vi "Datasheet Statistics Result.vi"(6 "Connection Refnum":T1, 8 "error in (no error)":errorcluster, 10 "Statistics Results":T3, 11 "Query Parameters":T5) -> (0 "error out":errorcluster, 1 "columns":i32, 2 "FORM":bool, 3 "Keyed Array":T2)   [LabVIEW 2011]
uses:
  Datasheet Analysis Parameters.ctl
  Statistics Data.ctl
  CGI SimpleStat Results.ctl
  ITK EXT/utils/keyedarr.llb/Keyed Array.ctl
  Summitek EXT/ODBC/SQL Controls/Connection Refnum.ctl
  ITK EXT/utils/strutil.llb/Case Matching.ctl
panel:
  out "Frequency Array":dbl[](array[numeric]) format="%#_14g"
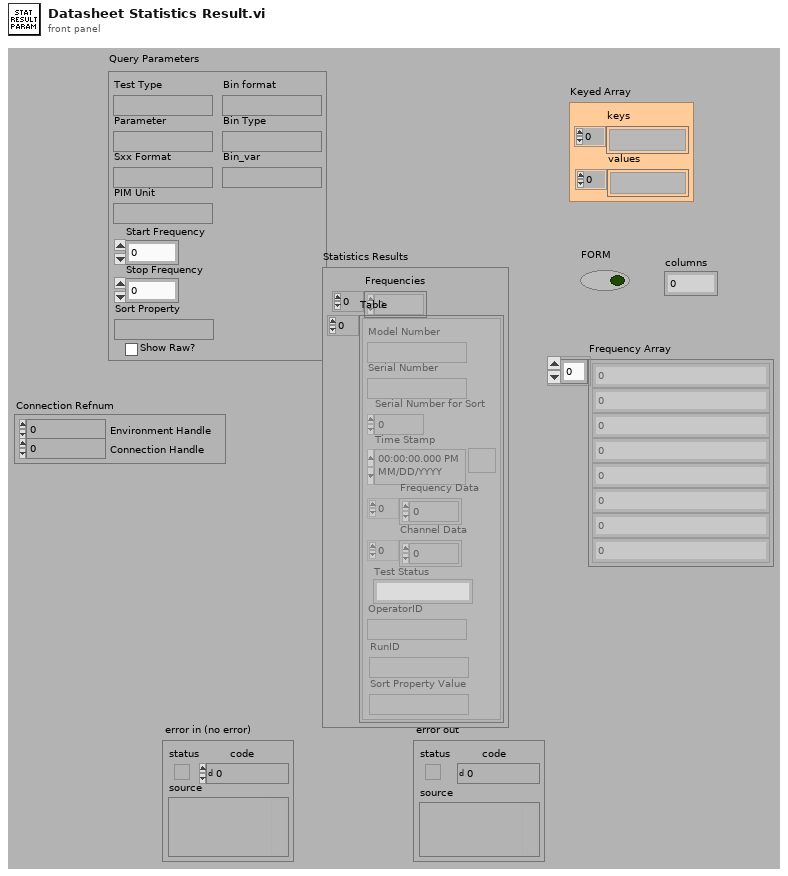
[diagram p1: front panel]
types:
  T1 = typedef "Connection Refnum.ctl" = cluster{"Environment Handle":i32, "Connection Handle":i32}
  T2 = typedef "Keyed Array.ctl" = cluster{"keys":string[], "values":string[]}
  T3 = typedef "Statistics Data.ctl" = cluster{"Table":T4[], "Frequencies":dbl[]}
  T4 = typedef "CGI SimpleStat Results.ctl" = cluster{"Model Number":string, "Serial Number for Sort":i32, "Serial Number":string, "Time Stamp":timestamp, "Channel Data":dbl[], "Test Status":string, "OperatorID":string, "Frequency Data":dbl[], "RunID":string, "Sort Property Value":string}
  T5 = typedef "Datasheet Analysis Parameters.ctl" = cluster{"Test Type":string, "Parameter":string, "Sxx Format":string, "PIM Unit":string, "Start Frequency":dbl, "Stop Frequency":dbl, "Sort Property":string, "Show Raw?":bool, "Bin format":string, "Bin Type":string, "Bin_var":string}
  T6 = typedef "Case Matching.ctl" = enum16{"a != A", "a == A", "system"}
  T7 = enum16{"Log MAG", "Lin MAG", "VSWR", "Phase", "Delay", "Insertion Loss", "Isolation", "Return Loss"}
  T8 = typedef "Field Record.ctl" = cluster{"ixField":i32, "iSequenceOrder":i32, "sxFieldId":string, "sxSequenceId":string, "sDisplayName":string, "sValue":string, "sUnits":string, "nDataType":T9, "nNextItem":T10, "fSystem":bool, "fSystemValue":bool, "fRequired":bool, "fSetAtTest":bool, "fTestField":bool, "fDeleted":bool, "fIndexed":bool, "fFreeList":bool}
  T9 = typedef "Field DataTypes.ctl" = enum32{"text", "numeric", "list", "timestamp", "boolean"}
  T10 = typedef "Field NextItem.ctl" = enum32{"Reset", "Retain", "Auto-Increment"}
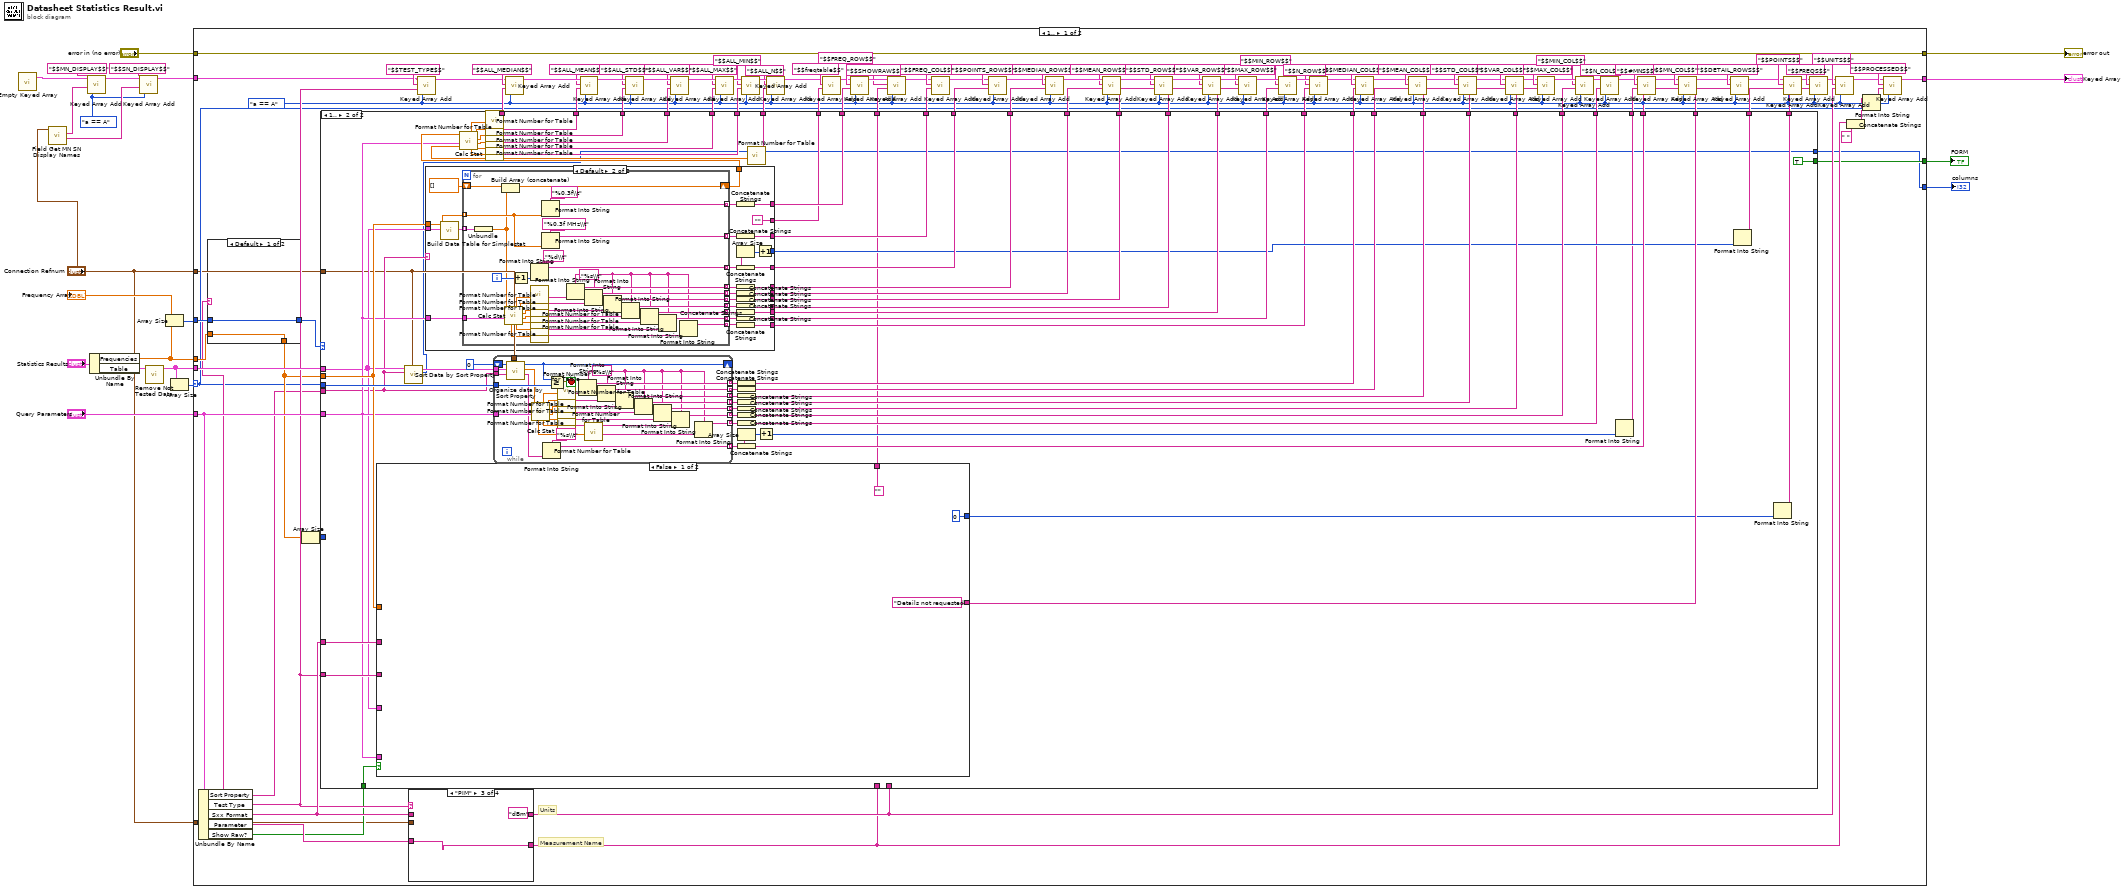
[diagram p0: block diagram]
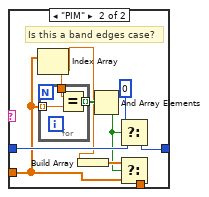
[diagram p2: hidden frame]
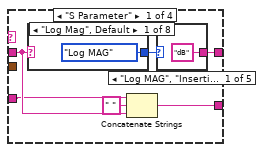
[diagram p3: hidden frame]
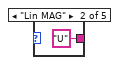
[diagram p4: hidden frame]
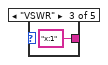
[diagram p5: hidden frame]
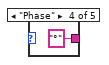
[diagram p6: hidden frame]
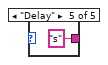
[diagram p7: hidden frame]
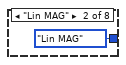
[diagram p8: hidden frame]
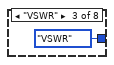
[diagram p9: hidden frame]
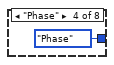
[diagram p10: hidden frame]
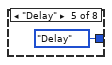
[diagram p11: hidden frame]
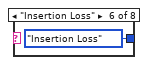
[diagram p12: hidden frame]
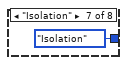
[diagram p13: hidden frame]
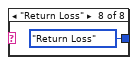
[diagram p14: hidden frame]
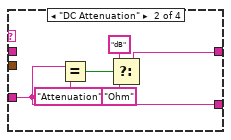
[diagram p15: hidden frame]
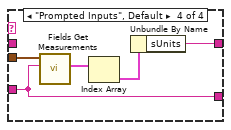
[diagram p16: hidden frame]
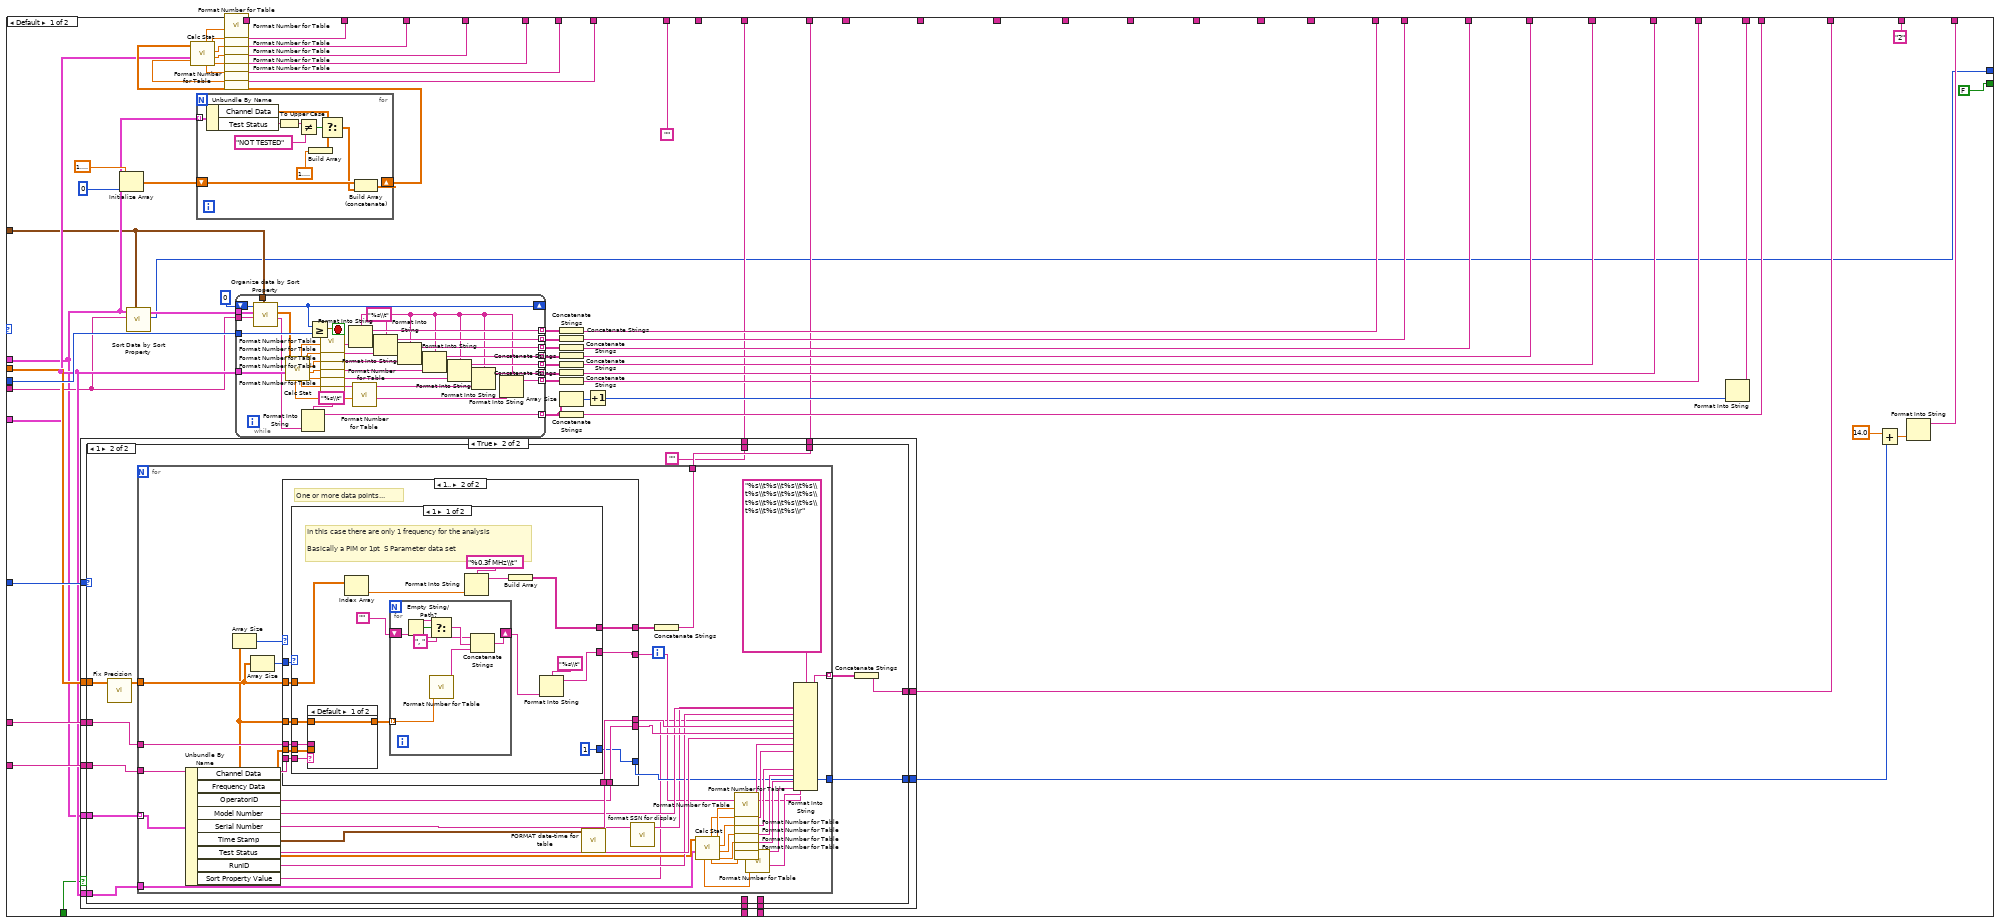
[diagram p17: hidden frame]
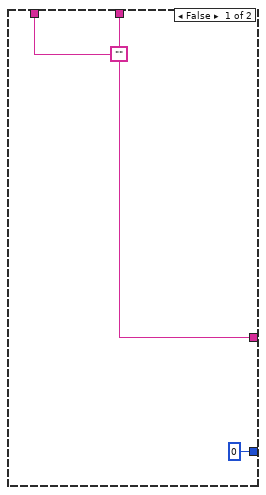
[diagram p18: hidden frame]
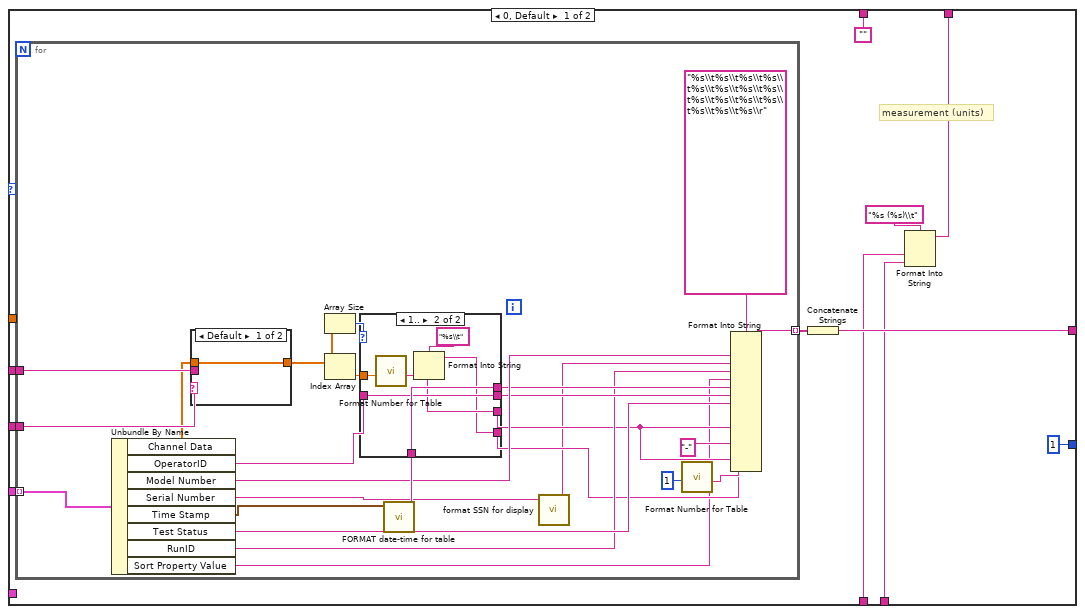
[diagram p19: hidden frame]
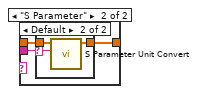
[diagram p20: hidden frame]
diagram:
  w5 = Case_Matching."a == A" ("case matching (sensitive)")
  n1 = call "Empty Keyed Array.vi"() -> ("empty keyed array"=w4:T2)  [unwired: 3 out]
  n2 = call "Field Get MN SN Display Names.vi"("Connection Refnum"="Connection Refnum") -> ("Serial Number Display Name"=w7:string, "Model Number Display Name"=w8:string)  [unwired: 1 in, 8 out]
  n3 = call "Keyed Array Add.vi"("case matching (sensitive)"=w5, "value"=w8, "key"="$$MN_DISPLAY$$", "array in"=w4) -> ("array out"=w9:T2)  [unwired: 3 out]
  n4 = Unbundle By Name("Statistics Results") -> ("Frequencies"=w15:dbl[], "Table"=w14:T4[])
  "Frequency Array" <- w15
  n5 = call "Keyed Array Add.vi"("case matching (sensitive)"=w5, "value"=w7, "key"="$$SN_DISPLAY$$", "array in"=w9) -> ("array out"=w6:T2)  [unwired: 3 out]
  n6 = call "Remove Not Tested Data.vi"("Table"=w14) -> ("Table 2"=w13:T4[])  [unwired: 10 out]
  n7 = Array Size(array=w15) -> (size(s)=w18:i32)
  n8 = Array Size(array=w13) -> (size(s)=w16:i32)
  n9 = case shown="1.." w16 {
    selector: w16 -> [w29 w775]
    tunnel: [w65 w801] -> w21
    tunnel: "error in (no error)" -> [w65 w801]
    tunnel: [w31 w777] -> w12
    tunnel: w18 -> [w61 w798]
    tunnel: "Query Parameters" -> [w130 w841]
    tunnel: w15 -> [w58 w797]
    tunnel: w13 -> [w131 _]
    tunnel: w6 -> [w35 w781]
    tunnel: "Connection Refnum" -> [w25 _]
    tunnel: "Connection Refnum" -> [w24 w770]
    tunnel: [w23 FALSE] -> w2
    tunnel: [w22 0] -> w1
    frame 1.. {
      w30 = Case_Matching."a == A" ("case matching (sensitive)")
      # "Measurement Name"
      # "Units"
      n10 = Unbundle By Name(w130) -> ("Sort Property"=w41:string, "Test Type"=w56:string, "Sxx Format"=w135:string, "Parameter"=w136:string, "Show Raw?"=w40:bool)
      n11 = case shown="Default" w56 {
        tunnel: w61 -> [w147 w156]
        tunnel: [w147 w155] -> w60
        tunnel: [w146 w152] -> w55
        tunnel: w58 -> [w146 w151]
        frame Default {
        }
        frame "PIM" {
          # "Is this a band edges case?"
          n12 = Index Array(array=w151) -> (element=w148:dbl)  [unwired: 1 in]
          n13 = for {
            tunnel: w148 -> [w159]
            tunnel: w151 -> [w158] mode=indexing
            tunnel: [w157] -> w150 mode=indexing
            n14 = Equal?(x=w159, y=w158) -> (x = y?=w157:bool)
          }
          n15 = Build Array(w148) -> (w153:dbl[])
          n16 = And Array Elements(Boolean array=w150) -> (logical AND=w149:bool)
          n17 = Select(t=0, s=w149, f=w156) -> (s? t:f=w155:i32)
          n18 = Select(t=w153, s=w149, f=w151) -> (s? t:f=w152:dbl[])
        }
      }
      n19 = Array Size(array=w55) -> (size(s)=w59:i32)
      n20 = case shown="\"PIM\"" w56 {
        tunnel: w135 -> [w162 _ _ _]
        tunnel: w136 -> [w160 w179 w185 w188]
        tunnel: [w164 w180 "dBm" ("search string") w189] -> w42
        tunnel: [w161 w179 w185 w188] -> w28
        tunnel: w24 -> [_ _ _ w187]
        frame "S Parameter" {
          n21 = case shown="\"Log Mag\", Default" w162 {
            tunnel: [T7."Log MAG" ("Display Format") T7."Lin MAG" ("Display Format") T7."VSWR" ("Display Format") T7."Phase" ("Display Format") T7."Delay" ("Display Format") T7."Insertion Loss" ("Display Format") T7."Isolation" ("Display Format") T7."Return Loss" ("Display Format")] -> w165
            frame "Log Mag", Default {
            }
            frame "Lin MAG" {
            }
            frame "VSWR" {
            }
            frame "Phase" {
            }
            frame "Delay" {
            }
            frame "Insertion Loss" {
            }
            frame "Isolation" {
            }
            frame "Return Loss" {
            }
          }
          n22 = Concatenate Strings(w160, " " ("search string"), w162) -> (w161:string)
          n23 = case shown="\"Log MAG\", \"Insertion Loss\"..\"Return Loss\", Default" w165 {
            tunnel: ["dB" "U" "x:1" "°" "s"] -> w164
            frame "Log MAG", "Insertion Loss".."Return Loss", Default {
            }
            frame "Lin MAG" {
            }
            frame "VSWR" {
            }
            frame "Phase" {
            }
            frame "Delay" {
            }
          }
        }
        frame "DC Attenuation" {
          n24 = Equal?(x=w179, y="Attenuation" ("search string")) -> (x = y?=w183:bool)
          n25 = Select(t="dB" ("search string"), s=w183, f="Ohm" ("search string")) -> (s? t:f=w180:string)
        }
        frame "PIM" {
        }
        frame "Prompted Inputs", Default {
          n26 = call "Fields Get Measurements.vi"("sDisplayName (empty, get all)"=w188, "Connection Refnum"=w187) -> ("Measurement Fields"=w191:T8[])  [unwired: 9 out]
          n27 = Index Array(array=w191) -> (element=w190:T8)  [unwired: 1 in]
          n28 = Unbundle By Name(w190) -> ("sUnits"=w189:string)
        }
      }
      n29 = case shown="1.." w60 {
        tunnel: w55 -> [w211 w506]
        tunnel: w131 -> [w198 w498]
        tunnel: w56 -> [w225 w551]
        tunnel: w135 -> [w226 w552]
        tunnel: w29 -> [w234 w553]
        tunnel: w130 -> [w210 w505]
        tunnel: [w233 w550] -> w129
        tunnel: [w232 w543] -> w128
        tunnel: [w231 w542] -> w125
        tunnel: [w229 w541] -> w124
        tunnel: [w228 w540] -> w123
        tunnel: [w227 w539] -> w122
        tunnel: [w230 w538] -> w121
        tunnel: [w247 w530] -> w107
        tunnel: [w246 w529] -> w106
        tunnel: [w245 w528] -> w105
        tunnel: [w244 w527] -> w104
        tunnel: [w243 w526] -> w103
        tunnel: [w242 w525] -> w102
        tunnel: [_ w524] -> w90
        tunnel: [_ w523] -> w89
        tunnel: [_ w522] -> w88
        tunnel: [_ w521] -> w87
        tunnel: [_ w520] -> w86
        tunnel: [_ w519] -> w85
        tunnel: [_ w518] -> w84
        tunnel: [_ w517] -> w82
        tunnel: [w224 w516] -> w77
        tunnel: w28 -> [w213 _]
        tunnel: [w208 w514] -> w71
        tunnel: ["2" w513] -> w70
        tunnel: [w220 w508] -> w67
        tunnel: ["" w494] -> w62
        tunnel: w59 -> [w214 _]
        tunnel: [w212 w507] -> w57
        tunnel: [w204 w503] -> w52
        tunnel: [_ w502] -> w47
        tunnel: [w202 w500] -> w44
        tunnel: w42 -> [w201 _]
        tunnel: w41 -> [w199 w495]
        tunnel: w40 -> [w197 w497]
        tunnel: [w196 w496] -> w37
        tunnel: w25 -> [w195 w493]
        tunnel: [FALSE TRUE] -> w23
        tunnel: [w192 w491] -> w22
        frame Default {
          n30 = case shown="True" w197 {
            tunnel: w226 -> [_ w267]
            tunnel: w225 -> [_ w266]
            tunnel: [w254 w265] -> w224
            tunnel: w214 -> [_ w264]
            tunnel: w213 -> [_ w263]
            tunnel: [w254 w262] -> w212
            tunnel: w211 -> [_ w261]
            tunnel: w210 -> [_ w260]
            tunnel: [0 w259] -> w206
            tunnel: w201 -> [_ w258]
            tunnel: w198 -> [_ w257]
            tunnel: [w254 w256] -> w196
            frame False {
              w254 = ""
            }
            frame True {
              n31 = case shown="1" w264 {
                tunnel: w257 -> [w278 w330]
                tunnel: w267 -> [w277 w328]
                tunnel: w266 -> [w276 w329]
                tunnel: [w274 w326] -> w265
                tunnel: w261 -> [_ w324]
                tunnel: [w272 w325] -> w262
                tunnel: w263 -> [w271 _]
                tunnel: w260 -> [_ w321]
                tunnel: [1 w322] -> w259
                tunnel: w258 -> [w269 _]
                tunnel: ["" ""] -> w256
                frame 0, Default {
                  # "measurement (units)"
                  n32 = for {
                    tunnel: w278 -> [w303] mode=indexing
                    tunnel: w276 -> [w298]
                    tunnel: w277 -> [w297]
                    tunnel: [w290] -> w275 mode=indexing
                    w287 = "-" ("search string")
                    n33 = Unbundle By Name(w303) -> ("Channel Data"=w296:dbl[], "OperatorID"=w295:string, "Model Number"=w293:string, "Serial Number"=w282:string, "Time Stamp"=w279:timestamp, "Test Status"=w294:string, "RunID"=w289:string, "Sort Property Value"=w280:string)
                    n34 = case shown="Default" w298 {
                      tunnel: [w304 w306] -> w299
                      tunnel: w297 -> [_ w305]
                      tunnel: w296 -> [w304 w307]
                      frame Default {
                      }
                      frame "S Parameter" {
                        n35 = case shown="Default" w305 {
                          selector: w305 -> [_ w309]
                          tunnel: w307 -> [w308 w311]
                          tunnel: [w308 w310] -> w306
                          frame "delay" {
                          }
                          frame Default {
                            n36 = call "S Parameter Unit Convert.vi"("Format"=w309, "Waveform IN"=w311) -> ("Waveform out"=w310:dbl[])  [unwired: 1 in, 8 out]
                          }
                        }
                      }
                    }
                    n37 = Array Size(array=w299) -> (size(s)=w302:i32)
                    n38 = Index Array(array=w299) -> (element=w301:dbl)  [unwired: 1 in]
                    n39 = call "FORMAT date-time for table.vi"("Time Stamp"=w279) -> ("String"=w300:string)  [unwired: 1 in, 9 out]
                    n40 = case shown="1.." w302 {
                      tunnel: [w312 w315] -> w284
                      tunnel: w301 -> [_ w317]
                      tunnel: w300 -> [_ w319]
                      tunnel: [w312 w319] -> w292
                      tunnel: [w312 w318] -> w291
                      tunnel: w295 -> [_ w318]
                      tunnel: ["Not Tested\\t" ("search string") w314] -> w283
                      frame 0, Default {
                        w312 = "-" ("search string")
                      }
                      frame 1.. {
                        n41 = call "Format Number for Table.vi"("Number"=w317) -> ("Number String"=w315:string)  [unwired: 2 in, 8 out]
                        n42 = Format Into String(format string="%s\\t", w315) -> (resulting string=w314:string)  [unwired: 2 in, 1 out]
                      }
                    }
                    n43 = call "format SSN for display.vi"("string"=w282) -> ("s? t:f"=w281:string)  [unwired: 4 out]
                    n44 = call "Format Number for Table.vi"("Number"=1) -> ("Number String"=w285:string)  [unwired: 2 in, 8 out]
                    n45 = Format Into String(format string="%s\\t%s\\t%s\\t%s\\t%s\\t%s\\t%s\\t%s\\t%s\\t%s\\t%s\\t%s\\t%s\\t%s\\t%s\\r", w293, w281, w289, w280, w292, w291, w294, w284, w284, w287, w287, w284, w284, w285, w283) -> (resulting string=w290:string)  [unwired: 2 in, 1 out]
                  }
                  n46 = Concatenate Strings(w275) -> (w274:string)
                  n47 = Format Into String(format string="%s (%s)\\t" ("search string"), w271, w269) -> (resulting string=w272:string)  [unwired: 2 in, 1 out]
                }
                frame 1 {
                  n48 = call "Fix Precision.vi"("DBL"=w324) -> ("DBLOut"=w323:dbl[])  [unwired: 10 out]
                  n49 = for {
                    tunnel: w330 -> [w370] mode=indexing
                    tunnel: w323 -> [w355]
                    tunnel: w329 -> [w367]
                    tunnel: w328 -> [w366]
                    tunnel: [w362] -> w327 mode=indexing
                    tunnel: [w339] -> w322
                    tunnel: [w357] -> w325
                    tunnel: w321 -> [w333]
                    n50 = Unbundle By Name(w370) -> ("Channel Data"=w346:dbl[], "Frequency Data"=w361:dbl[], "OperatorID"=w359:string, "Model Number"=w360:string, "Serial Number"=w335:string, "Time Stamp"=w331:timestamp, "Test Status"=w363:string, "RunID"=w358:string, "Sort Property Value"=w332:string)
                    n51 = Array Size(array=w346) -> (size(s)=w369:i32)
                    n52 = Array Size(array=w355) -> (size(s)=w354:i32)
                    n53 = call "FORMAT date-time for table.vi"("Time Stamp"=w331) -> ("String"=w368:string)  [unwired: 1 in, 9 out]
                    n54 = case shown="1.." w369 {
                      tunnel: w346 -> [_ w389]
                      tunnel: ["Not Tested" ("search string") w390] -> w365
                      tunnel: w368 -> [_ w390]
                      tunnel: w355 -> [w376 w383]
                      tunnel: w367 -> [_ w388]
                      tunnel: w366 -> [_ w387]
                      tunnel: w359 -> [_ w386]
                      tunnel: [w374 w386] -> w364
                      tunnel: w361 -> [_ w385]
                      tunnel: [_ w384] -> w356
                      tunnel: w354 -> [_ w382]
                      tunnel: [w373 w381] -> w336
                      tunnel: [w371 w380] -> w339
                      frame Default {
                        w374 = "-" ("search string")
                        # "This is no data case"
                        n55 = for {
                          tunnel: w376 -> [_] mode=indexing
                          tunnel: w374 -> [w377]
                          tunnel: [w378] -> w372 mode=indexing
                          n56 = Format Into String(format string="%s\\t", w377) -> (resulting string=w378:string)  [unwired: 2 in, 1 out]
                        }
                        n57 = Array Size(array=w372) -> (size(s)=w371:i32)
                        n58 = Concatenate Strings(w372) -> (w373:string)
                      }
                      frame 1.. {
                        # "One or more data points..."
                        n59 = case shown="1" w382 {
                          tunnel: w389 -> [w405 w428]
                          tunnel: w388 -> [w404 w427]
                          tunnel: w387 -> [w403 w426]
                          tunnel: w385 -> [w402 w422]
                          tunnel: [w397 w425] -> w384
                          tunnel: w383 -> [w400 w423]
                          tunnel: [w396 w420] -> w381
                          tunnel: [1 w418] -> w380
                          frame 1 {
                            # "In this case there are only 1 frequency for the analysis   \n\nBasically a PIM or 1pt  S Parameter data set"
                            n60 = case shown="Default" w404 {
                              tunnel: w405 -> [w413 w417]
                              tunnel: [w413 w416] -> w393
                              tunnel: w403 -> [_ w415]
                              tunnel: w402 -> [_ w414]
                              frame Default {
                              }
                              frame "S Parameter" {
                                n61 = call "S Parameter Unit Convert.vi"("Frequency Array"=w414, "Format"=w415, "Waveform IN"=w417) -> ("Waveform out"=w416:dbl[])  [unwired: 8 out]
                              }
                            }
                            n62 = Index Array(array=w400) -> (element=w399:dbl)  [unwired: 1 in]
                            n63 = for {
                              shift-right: [w411] -> w392
                              shift-left: "" -> [w407]
                              tunnel: w393 -> [w406] mode=indexing
                              n64 = Empty String/Path?(string/path=w407) -> (empty?=w410:bool)
                              n65 = Select(t=w407, s=w410, f=", " ("format string")) -> (s? t:f=w408:string)
                              n66 = call "Format Number for Table.vi"("Number"=w406) -> ("Number String"=w412:string)  [unwired: 2 in, 8 out]
                              n67 = Concatenate Strings(w407, w408, w412) -> (w411:string)
                            }
                            n68 = Format Into String(format string="%0.3f MHz\\t" ("search string"), w399) -> (resulting string=w398:string)  [unwired: 2 in, 1 out]
                            n69 = Build Array(w398) -> (w397:string[])
                            n70 = Format Into String(format string="%s\\t", w392) -> (resulting string=w396:string)  [unwired: 2 in, 1 out]
                          }
                          frame Default {
                            # "For this case, like PI.weight.  There are no Frequencies"
                            n71 = case shown="Default" w427 {
                              tunnel: w428 -> [w429 w433]
                              tunnel: [w429 w432] -> w424
                              tunnel: w426 -> [_ w431]
                              tunnel: w422 -> [_ w430]
                              frame Default {
                              }
                              frame "S Parameter" {
                                n72 = call "S Parameter Unit Convert.vi"("Frequency Array"=w430, "Format"=w431, "Waveform IN"=w433) -> ("Waveform out"=w432:dbl[])  [unwired: 8 out]
                              }
                            }
                            n73 = call "Fix Precision.vi"("DBL"=w422) -> ("DBLOut"=w421:dbl[])  [unwired: 10 out]
                            n74 = for {
                              tunnel: [w439] -> w419 mode=indexing
                              tunnel: w423 -> [w435] mode=indexing
                              tunnel: w421 -> [_]
                              tunnel: w424 -> [w444]
                              tunnel: [w434] -> w425 mode=indexing
                              i -> [w437]
                              n75 = Less Than 0?(x=w437) -> (x < 0?=w445:bool)
                              n76 = Index Array(array=w444, index=w437) -> (element=w443:dbl)
                              n77 = Select(t=1.1447298858494002, s=w445, f=w443) -> (s? t:f=w442:dbl)
                              n78 = Format Into String(format string="%0.3f MHz\\t" ("search string"), w435) -> (resulting string=w434:string)  [unwired: 2 in, 1 out]
                              n79 = call "Format Number for Table.vi"("Number"=w442) -> ("Number String"=w440:string)  [unwired: 2 in, 8 out]
                              n80 = Format Into String(format string="%s\\t", w440) -> (resulting string=w439:string)  [unwired: 2 in, 1 out]
                            }
                            n81 = Concatenate Strings(w419) -> (w420:string)
                            n82 = Array Size(array=w419) -> (size(s)=w418:i32)
                          }
                        }
                      }
                    }
                    n83 = call "format SSN for display.vi"("string"=w335) -> ("s? t:f"=w334:string)  [unwired: 4 out]
                    n84 = Concatenate Strings(w356) -> (w357:string)
                    n85 = call "Calc Stat.vi"("Query Parameters"=w333, "Channel Data"=w346) -> ("Maximum"=w348:dbl, "Variance"=w349:dbl, "Standard Deviation"=w350:dbl, "Mean"=w352:dbl, "Minimum"=w347:dbl, "Median"=w351:dbl, "N"=w338:dbl)  [unwired: 2 in, 1 out]
                    n86 = call "Format Number for Table.vi"("Number"=w352) -> ("Number String"=w345:string)  [unwired: 2 in, 8 out]
                    n87 = call "Format Number for Table.vi"("Number"=w351) -> ("Number String"=w344:string)  [unwired: 2 in, 8 out]
                    n88 = call "Format Number for Table.vi"("Number"=w350) -> ("Number String"=w343:string)  [unwired: 2 in, 8 out]
                    n89 = call "Format Number for Table.vi"("Number"=w349) -> ("Number String"=w342:string)  [unwired: 2 in, 8 out]
                    n90 = call "Format Number for Table.vi"("Number"=w348) -> ("Number String"=w341:string)  [unwired: 2 in, 8 out]
                    n91 = call "Format Number for Table.vi"("Number"=w347) -> ("Number String"=w340:string)  [unwired: 2 in, 8 out]
                    n92 = call "Format Number for Table.vi"("Number"=w338) -> ("Number String"=w337:string)  [unwired: 2 in, 8 out]
                    n93 = Format Into String(format string="%s\\t%s\\t%s\\t%s\\t%s\\t%s\\t%s\\t%s\\t%s\\t%s\\t%s\\t%s\\t%s\\t%s\\t%s\\r", w360, w334, w358, w332, w365, w364, w363, w345, w344, w343, w342, w341, w340, w337, w336) -> (resulting string=w362:string)  [unwired: 2 in, 1 out]
                  }
                  n94 = Concatenate Strings(w327) -> (w326:string)
                }
              }
            }
          }
          n95 = Initialize Array(1.1447298858494002, 0 ("dimension size")) -> (w218:dbl[])
          n96 = call "Sort Data by Sort Property.vi"("Connection Refnum"=w195, "Sort Property Name"=w199, "Table"=w198) -> ("Numeric"=w192:i32, "Table 2"=w200:T4[])  [unwired: 1 in, 6 out]
          n97 = for {
            tunnel: w198 -> [w490] mode=indexing
            shift-right: [w482] -> w215
            shift-left: w218 -> [w484]
            n98 = Unbundle By Name(w490) -> ("Channel Data"=w487:dbl[], "Test Status"=w489:string)
            n99 = To Upper Case(1:w489) -> (0:w480:string)
            n100 = Not Equal?(x=w480, y="NOT TESTED" ("key")) -> (x != y?=w488:bool)
            n101 = Build Array(1.1447298858494002) -> (w486:dbl[])
            n102 = Select(t=w487, s=w488, f=w486) -> (s? t:f=w483:dbl[])
            n103 = Build Array (concatenate)(w484, w483) -> (w482:dbl[])
          }
          n104 = call "Calc Stat.vi"("Query Parameters"=w210, "Channel Data"=w215) -> ("Maximum"=w248:dbl, "Variance"=w250:dbl, "Standard Deviation"=w251:dbl, "Mean"=w252:dbl, "Minimum"=w249:dbl, "Median"=w253:dbl, "N"=w205:dbl)  [unwired: 2 in, 1 out]
          n105 = call "Format Number for Table.vi"("Number"=w253) -> ("Number String"=w247:string)  [unwired: 2 in, 8 out]
          n106 = call "Format Number for Table.vi"("Number"=w252) -> ("Number String"=w246:string)  [unwired: 2 in, 8 out]
          n107 = call "Format Number for Table.vi"("Number"=w251) -> ("Number String"=w245:string)  [unwired: 2 in, 8 out]
          n108 = call "Format Number for Table.vi"("Number"=w250) -> ("Number String"=w244:string)  [unwired: 2 in, 8 out]
          n109 = call "Format Number for Table.vi"("Number"=w248) -> ("Number String"=w243:string)  [unwired: 2 in, 8 out]
          n110 = call "Format Number for Table.vi"("Number"=w249) -> ("Number String"=w242:string)  [unwired: 2 in, 8 out]
          n111 = call "Format Number for Table.vi"("Number"=w205) -> ("Number String"=w204:string)  [unwired: 2 in, 8 out]
          n112 = while {
            shift-right: [w446] -> _
            shift-left: 0 -> [w479]
            tunnel: w200 -> [w478]
            tunnel: w234 -> [w477]
            tunnel: w210 -> [w474]
            tunnel: [w465] -> w221 mode=indexing
            tunnel: [w463] -> w240 mode=indexing
            tunnel: [w457] -> w239 mode=indexing
            tunnel: [w456] -> w238 mode=indexing
            tunnel: [w455] -> w237 mode=indexing
            tunnel: [w454] -> w236 mode=indexing
            tunnel: [w453] -> w235 mode=indexing
            tunnel: [w449] -> w203 mode=indexing
            tunnel: w199 -> [w448]
            tunnel: w195 -> [w447]
            stop <- w476 stop-if-true
            w452 = "%s\\t" ("format string")
            n113 = call "Organize data by Sort Property.vi"("Connection Refnum"=w447, "Sort Property Name"=w448, "Table"=w478, "Start Index"=w479) -> ("Property Value"=w467:string, "Channel Data"=w475:dbl[], "End Index"=w446:i32)  [unwired: 1 in, 4 out]
            n114 = call "Calc Stat.vi"("Query Parameters"=w474, "Channel Data"=w475) -> ("Maximum"=w473:dbl, "Variance"=w471:dbl, "Standard Deviation"=w470:dbl, "Mean"=w469:dbl, "Minimum"=w472:dbl, "Median"=w468:dbl, "N"=w451:dbl)  [unwired: 2 in, 1 out]
            n115 = Format Into String(format string="%s\\t", w467) -> (resulting string=w465:string)  [unwired: 2 in, 1 out]
            n116 = Greater Or Equal?(x=w446, y=w477) -> (x >= y?=w476:bool)
            n117 = call "Format Number for Table.vi"("Number"=w468) -> ("Number String"=w464:string)  [unwired: 2 in, 8 out]
            n118 = call "Format Number for Table.vi"("Number"=w469) -> ("Number String"=w462:string)  [unwired: 2 in, 8 out]
            n119 = call "Format Number for Table.vi"("Number"=w470) -> ("Number String"=w461:string)  [unwired: 2 in, 8 out]
            n120 = call "Format Number for Table.vi"("Number"=w471) -> ("Number String"=w460:string)  [unwired: 2 in, 8 out]
            n121 = call "Format Number for Table.vi"("Number"=w473) -> ("Number String"=w459:string)  [unwired: 2 in, 8 out]
            n122 = call "Format Number for Table.vi"("Number"=w472) -> ("Number String"=w458:string)  [unwired: 2 in, 8 out]
            n123 = Format Into String(format string=w452, w464) -> (resulting string=w463:string)  [unwired: 2 in, 1 out]
            n124 = call "Format Number for Table.vi"("Number"=w451) -> ("Number String"=w450:string)  [unwired: 2 in, 8 out]
            n125 = Format Into String(format string=w452, w462) -> (resulting string=w457:string)  [unwired: 2 in, 1 out]
            n126 = Format Into String(format string=w452, w461) -> (resulting string=w456:string)  [unwired: 2 in, 1 out]
            n127 = Format Into String(format string=w452, w460) -> (resulting string=w455:string)  [unwired: 2 in, 1 out]
            n128 = Format Into String(format string=w452, w459) -> (resulting string=w454:string)  [unwired: 2 in, 1 out]
            n129 = Format Into String(format string=w452, w458) -> (resulting string=w453:string)  [unwired: 2 in, 1 out]
            n130 = Format Into String(format string=w452, w450) -> (resulting string=w449:string)  [unwired: 2 in, 1 out]
          }
          n131 = Concatenate Strings(w240) -> (w232:string)
          n132 = Concatenate Strings(w239) -> (w231:string)
          n133 = Concatenate Strings(w238) -> (w230:string)
          n134 = Concatenate Strings(w237) -> (w229:string)
          n135 = Concatenate Strings(w236) -> (w228:string)
          n136 = Concatenate Strings(w235) -> (w227:string)
          n137 = Concatenate Strings(w203) -> (w202:string)
          n138 = Array Size(array=w221) -> (size(s)=w222:i32)
          n139 = Concatenate Strings(w221) -> (w233:string)
          n140 = Increment(x=w222) -> (x+1=w219:i32)
          n141 = Format Into String(w219) -> (resulting string=w220:string)  [unwired: 3 in, 1 out]
          n142 = Add(x=14.0, y=w206) -> (x+y=w209:dbl)
          n143 = Format Into String(w209) -> (resulting string=w208:string)  [unwired: 3 in, 1 out]
        }
        frame 1.. {
          n144 = case shown="False" w497 {
            tunnel: w552 -> [_ w643]
            tunnel: w551 -> [_ w642]
            tunnel: ["Details not requested" w640] -> w516
            tunnel: [0 w637] -> w515
            tunnel: w506 -> [_ w636]
            tunnel: w505 -> [_ w635]
            tunnel: w498 -> [_ w634]
            tunnel: ["" ""] -> w496
            frame False {
            }
            frame True {
              n145 = for {
                tunnel: w634 -> [w682] mode=indexing
                tunnel: w636 -> [w654]
                tunnel: w642 -> [w679]
                tunnel: w643 -> [w678]
                tunnel: [w673] -> w641 mode=indexing
                tunnel: [w669] -> w639
                tunnel: w635 -> [w667]
                # "ALL Frequency"
                # "P/F"
                # "Operator"
                # "time"
                # "Run"
                # "SN"
                # "MN"
                # "Need to extract array that represents the repeated points in the PIM sweep\nand show the maximum."
                n146 = Unbundle By Name(w682) -> ("Channel Data"=w668:dbl[], "Frequency Data"=w672:dbl[], "OperatorID"=w671:string, "Model Number"=w648:string, "Serial Number"=w649:string, "Time Stamp"=w644:timestamp, "Test Status"=w674:string, "RunID"=w646:string, "Sort Property Value"=w645:string)
                n147 = call "Fix Precision.vi"("DBL"=w654) -> ("DBLOut"=w653:dbl[])  [unwired: 10 out]
                n148 = Array Size(array=w668) -> (size(s)=w681:i32)
                n149 = call "FORMAT date-time for table.vi"("Time Stamp"=w644) -> ("String"=w680:string)  [unwired: 1 in, 9 out]
                n150 = case shown="1.." w681 {
                  tunnel: w668 -> [_ w697]
                  tunnel: [w685 w699] -> w670
                  tunnel: ["Not Tested" ("search string") w698] -> w676
                  tunnel: w680 -> [_ w698]
                  tunnel: w653 -> [w686 w693]
                  tunnel: w679 -> [_ w696]
                  tunnel: w678 -> [_ w695]
                  tunnel: w671 -> [_ w694]
                  tunnel: [w683 w694] -> w675
                  tunnel: w672 -> [_ w691]
                  frame 0, Default {
                    w683 = "-" ("search string")
                    n151 = for {
                      tunnel: w686 -> [_] mode=indexing
                      tunnel: w683 -> [w687]
                      tunnel: [w688] -> w685 mode=indexing
                      n152 = Format Into String(format string="%s\\t", w687) -> (resulting string=w688:string)  [unwired: 2 in, 1 out]
                    }
                  }
                  frame 1.. {
                    n153 = case shown="\"S Parameter\"" w696 {
                      tunnel: w697 -> [w700 w704]
                      tunnel: [w700 w703] -> w692
                      tunnel: w695 -> [_ w702]
                      tunnel: w691 -> [_ w701]
                      frame Default {
                      }
                      frame "S Parameter" {
                        n154 = call "S Parameter Unit Convert.vi"("Frequency Array"=w701, "Format"=w702, "Waveform IN"=w704) -> ("Waveform out"=w703:dbl[])  [unwired: 8 out]
                      }
                    }
                    n155 = call "Fix Precision.vi"("DBL"=w691) -> ("DBLOut"=w690:dbl[])  [unwired: 10 out]
                    n156 = for {
                      tunnel: [w708] -> w699 mode=indexing
                      tunnel: w693 -> [w711] mode=indexing
                      tunnel: w690 -> [w712]
                      tunnel: w692 -> [w710]
                      n157 = while {
                        tunnel: w712 -> [w728]
                        tunnel: w711 -> [w727]
                        tunnel: w710 -> [w726]
                        shift-right: [w720] -> _
                        shift-left: 0 -> [w722]
                        shift-right: [w718] -> w705
                        shift-left: "" -> [w714]
                        stop <- w713 stop-if-true
                        n158 = Empty String/Path?(string/path=w714) -> (empty?=w717:bool)
                        n159 = Search 1D Array(1D array=w728, element=w727, start index (0)=w722) -> (index of element=w721:i32)
                        n160 = Less Than 0?(x=w721) -> (x < 0?=w713:bool)
                        n161 = Select(t=w714, s=w717, f=", " ("format string")) -> (s? t:f=w715:string)
                        n162 = Index Array(array=w726, index=w721) -> (element=w725:dbl)
                        n163 = Select(t=1.1447298858494002, s=w713, f=w725) -> (s? t:f=w724:dbl)
                        n164 = Increment(x=w721) -> (x+1=w720:i32)
                        n165 = call "Format Number for Table.vi"("Number"=w724) -> ("Number String"=w719:string)  [unwired: 2 in, 8 out]
                        n166 = case shown="True" w713 {
                          tunnel: w719 -> [w732 _]
                          tunnel: [w731 w733] -> w718
                          tunnel: w715 -> [w730 _]
                          tunnel: w714 -> [w729 w733]
                          frame False {
                            n167 = Concatenate Strings(w729, w730, w732) -> (w731:string)
                          }
                          frame True {
                          }
                        }
                      }
                      n168 = Format Into String(format string="%s\\t", w705) -> (resulting string=w708:string)  [unwired: 2 in, 1 out]
                    }
                  }
                }
                n169 = call "format SSN for display.vi"("string"=w649) -> ("s? t:f"=w647:string)  [unwired: 4 out]
                n170 = Array Size(array=w670) -> (size(s)=w669:i32)
                n171 = Concatenate Strings(w670) -> (w651:string)
                n172 = call "Calc Stat.vi"("Query Parameters"=w667, "Channel Data"=w668) -> ("Maximum"=w658:dbl, "Variance"=w660:dbl, "Standard Deviation"=w662:dbl, "Mean"=w666:dbl, "Minimum"=w656:dbl, "Median"=w664:dbl, "N"=w652:dbl)  [unwired: 2 in, 1 out]
                n173 = call "Format Number for Table.vi"("Number"=w666) -> ("Number String"=w665:string)  [unwired: 2 in, 8 out]
                n174 = call "Format Number for Table.vi"("Number"=w664) -> ("Number String"=w663:string)  [unwired: 2 in, 8 out]
                n175 = call "Format Number for Table.vi"("Number"=w662) -> ("Number String"=w661:string)  [unwired: 2 in, 8 out]
                n176 = call "Format Number for Table.vi"("Number"=w660) -> ("Number String"=w659:string)  [unwired: 2 in, 8 out]
                n177 = call "Format Number for Table.vi"("Number"=w658) -> ("Number String"=w657:string)  [unwired: 2 in, 8 out]
                n178 = call "Format Number for Table.vi"("Number"=w656) -> ("Number String"=w655:string)  [unwired: 2 in, 8 out]
                n179 = call "Format Number for Table.vi"("Number"=w652) -> ("Number String"=w650:string)  [unwired: 2 in, 8 out]
                n180 = Format Into String(format string="%s\\t%s\\t%s\\t%s\\t%s\\t%s\\t%s\\t%s\\t%s\\t%s\\t%s\\t%s\\t%s\\t%s\\t%s\\r", w648, w647, w646, w645, w676, w675, w674, w665, w663, w661, w659, w657, w655, w650, w651) -> (resulting string=w673:string)  [unwired: 2 in, 1 out]
              }
              n181 = Add(x=w639, y=14) -> (x+y=w637:i32)
              n182 = Concatenate Strings(w641) -> (w640:string)
            }
          }
          n183 = call "Sort Data by Sort Property.vi"("Connection Refnum"=w493, "Sort Property Name"=w495, "Table"=w498) -> ("Numeric"=w491:i32, "Table 2"=w499:T4[])  [unwired: 1 in, 6 out]
          n184 = case shown="Default" w495 {
            tunnel: [w561 w592] -> w531
            tunnel: [w555 w585] -> w524
            tunnel: [w555 w584] -> w523
            tunnel: [w555 w583] -> w522
            tunnel: [w555 w582] -> w521
            tunnel: [w555 w581] -> w520
            tunnel: [w555 w580] -> w519
            tunnel: [w555 w578] -> w518
            tunnel: [w555 w577] -> w517
            tunnel: [w559 w574] -> w512
            tunnel: [w557 w572] -> w507
            tunnel: w506 -> [w558 w571]
            tunnel: w505 -> [_ w569]
            tunnel: [w555 w567] -> w502
            tunnel: w498 -> [_ w566]
            tunnel: [w555 ""] -> w494
            frame "SPARA" {
              w559 = 0 ("dimension size")
              w555 = ""
              n185 = for {
                tunnel: w558 -> [w563] mode=indexing
                tunnel: [w562] -> w556 mode=indexing
                n186 = Format Into String(format string="%0.3f MHz\\t" ("search string"), w563) -> (resulting string=w562:string)  [unwired: 2 in, 1 out]
              }
              n187 = Initialize Array(0.0 ("dimension size"), w559) -> (w561:dbl[])
              n188 = Concatenate Strings(w556) -> (w557:string)
            }
            frame Default {
              n189 = call "Build Data Table for Simplestat.vi"("Table"=w566, "Frequency Array"=w571) -> ("All Data by Frequency"=w570:cluster{"Array":dbl[]}[])  [unwired: 1 in, 8 out]
              n190 = for {
                tunnel: w571 -> [w629] mode=indexing
                tunnel: [w624] -> w576 mode=indexing
                tunnel: w569 -> [w615]
                tunnel: [w622] -> w579 mode=indexing
                tunnel: [w623] -> w575 mode=indexing
                shift-right: [w625] -> w592
                shift-left: dbl[] [] -> [w626]
                tunnel: [w605] -> w591 mode=indexing
                tunnel: [w604] -> w590 mode=indexing
                tunnel: [w603] -> w589 mode=indexing
                tunnel: [w602] -> w588 mode=indexing
                tunnel: [w601] -> w587 mode=indexing
                tunnel: [w600] -> w586 mode=indexing
                tunnel: w570 -> [w599] mode=indexing
                tunnel: [w594] -> w568 mode=indexing
                i -> [w612]
                w597 = "%s\\t" ("format string")
                n191 = Unbundle(w599) -> ("Array"=w598:dbl[])
                n192 = Build Array (concatenate)(w626, w598) -> (w625:dbl[])
                n193 = call "Calc Stat.vi"("Query Parameters"=w615, "Channel Data"=w598) -> ("Maximum"=w616:dbl, "Variance"=w618:dbl, "Standard Deviation"=w619:dbl, "Mean"=w620:dbl, "Minimum"=w617:dbl, "Median"=w621:dbl, "N"=w595:dbl)  [unwired: 2 in, 1 out]
                n194 = Increment(x=w612) -> (x+1=w627:i32)
                n195 = Format Into String(format string="%d\\t" ("search string"), w627) -> (resulting string=w623:string)  [unwired: 2 in, 1 out]
                n196 = call "Format Number for Table.vi"("Number"=w621) -> ("Number String"=w611:string)  [unwired: 2 in, 8 out]
                n197 = call "Format Number for Table.vi"("Number"=w620) -> ("Number String"=w610:string)  [unwired: 2 in, 8 out]
                n198 = call "Format Number for Table.vi"("Number"=w619) -> ("Number String"=w609:string)  [unwired: 2 in, 8 out]
                n199 = call "Format Number for Table.vi"("Number"=w618) -> ("Number String"=w608:string)  [unwired: 2 in, 8 out]
                n200 = call "Format Number for Table.vi"("Number"=w616) -> ("Number String"=w607:string)  [unwired: 2 in, 8 out]
                n201 = call "Format Number for Table.vi"("Number"=w617) -> ("Number String"=w606:string)  [unwired: 2 in, 8 out]
                n202 = call "Format Number for Table.vi"("Number"=w595) -> ("Number String"=w596:string)  [unwired: 2 in, 8 out]
                n203 = Format Into String(format string="%0.3f\\t" ("search string"), w629) -> (resulting string=w622:string)  [unwired: 2 in, 1 out]
                n204 = Format Into String(format string="%0.3f MHz\\t" ("search string"), w629) -> (resulting string=w624:string)  [unwired: 2 in, 1 out]
                n205 = Format Into String(format string=w597, w611) -> (resulting string=w605:string)  [unwired: 2 in, 1 out]
                n206 = Format Into String(format string=w597, w610) -> (resulting string=w604:string)  [unwired: 2 in, 1 out]
                n207 = Format Into String(format string=w597, w609) -> (resulting string=w603:string)  [unwired: 2 in, 1 out]
                n208 = Format Into String(format string=w597, w608) -> (resulting string=w602:string)  [unwired: 2 in, 1 out]
                n209 = Format Into String(format string=w597, w607) -> (resulting string=w601:string)  [unwired: 2 in, 1 out]
                n210 = Format Into String(format string=w597, w606) -> (resulting string=w600:string)  [unwired: 2 in, 1 out]
                n211 = Format Into String(format string=w597, w596) -> (resulting string=w594:string)  [unwired: 2 in, 1 out]
              }
              n212 = Concatenate Strings(w579) -> (w578:string)
              n213 = Concatenate Strings(w576) -> (w572:string)
              n214 = Array Size(array=w575) -> (size(s)=w573:i32)
              n215 = Concatenate Strings(w575) -> (w577:string)
              n216 = Concatenate Strings(w591) -> (w585:string)
              n217 = Concatenate Strings(w590) -> (w584:string)
              n218 = Concatenate Strings(w589) -> (w583:string)
              n219 = Concatenate Strings(w588) -> (w582:string)
              n220 = Concatenate Strings(w587) -> (w581:string)
              n221 = Concatenate Strings(w586) -> (w580:string)
              n222 = Concatenate Strings(w568) -> (w567:string)
              n223 = Increment(x=w573) -> (x+1=w574:i32)
            }
          }
          n224 = call "Calc Stat.vi"("Query Parameters"=w505, "Channel Data"=w531) -> ("Maximum"=w532:dbl, "Variance"=w534:dbl, "Standard Deviation"=w535:dbl, "Mean"=w536:dbl, "Minimum"=w533:dbl, "Median"=w537:dbl, "N"=w504:dbl)  [unwired: 2 in, 1 out]
          n225 = call "Format Number for Table.vi"("Number"=w537) -> ("Number String"=w530:string)  [unwired: 2 in, 8 out]
          n226 = call "Format Number for Table.vi"("Number"=w536) -> ("Number String"=w529:string)  [unwired: 2 in, 8 out]
          n227 = call "Format Number for Table.vi"("Number"=w535) -> ("Number String"=w528:string)  [unwired: 2 in, 8 out]
          n228 = call "Format Number for Table.vi"("Number"=w534) -> ("Number String"=w527:string)  [unwired: 2 in, 8 out]
          n229 = call "Format Number for Table.vi"("Number"=w532) -> ("Number String"=w526:string)  [unwired: 2 in, 8 out]
          n230 = call "Format Number for Table.vi"("Number"=w533) -> ("Number String"=w525:string)  [unwired: 2 in, 8 out]
          n231 = while {
            shift-right: [w735] -> _
            shift-left: 0 -> [w767]
            tunnel: w499 -> [w766]
            tunnel: w553 -> [w765]
            tunnel: w505 -> [w762]
            tunnel: [w753] -> w510 mode=indexing
            tunnel: [w751] -> w549 mode=indexing
            tunnel: [w745] -> w548 mode=indexing
            tunnel: [w744] -> w547 mode=indexing
            tunnel: [w743] -> w546 mode=indexing
            tunnel: [w742] -> w545 mode=indexing
            tunnel: [w741] -> w544 mode=indexing
            tunnel: [w737] -> w501 mode=indexing
            tunnel: w495 -> [w736]
            tunnel: w493 -> [w734]
            stop <- w764 stop-if-true
            w740 = "%s\\t" ("format string")
            n232 = call "Organize data by Sort Property.vi"("Connection Refnum"=w734, "Sort Property Name"=w736, "Table"=w766, "Start Index"=w767) -> ("Property Value"=w755:string, "Channel Data"=w763:dbl[], "End Index"=w735:i32)  [unwired: 1 in, 4 out]
            n233 = call "Calc Stat.vi"("Query Parameters"=w762, "Channel Data"=w763) -> ("Maximum"=w761:dbl, "Variance"=w759:dbl, "Standard Deviation"=w758:dbl, "Mean"=w757:dbl, "Minimum"=w760:dbl, "Median"=w756:dbl, "N"=w739:dbl)  [unwired: 2 in, 1 out]
            n234 = Format Into String(format string="%s\\t", w755) -> (resulting string=w753:string)  [unwired: 2 in, 1 out]
            n235 = Greater Or Equal?(x=w735, y=w765) -> (x >= y?=w764:bool)
            n236 = call "Format Number for Table.vi"("Number"=w756) -> ("Number String"=w752:string)  [unwired: 2 in, 8 out]
            n237 = call "Format Number for Table.vi"("Number"=w757) -> ("Number String"=w750:string)  [unwired: 2 in, 8 out]
            n238 = call "Format Number for Table.vi"("Number"=w758) -> ("Number String"=w749:string)  [unwired: 2 in, 8 out]
            n239 = call "Format Number for Table.vi"("Number"=w759) -> ("Number String"=w748:string)  [unwired: 2 in, 8 out]
            n240 = call "Format Number for Table.vi"("Number"=w761) -> ("Number String"=w747:string)  [unwired: 2 in, 8 out]
            n241 = call "Format Number for Table.vi"("Number"=w760) -> ("Number String"=w746:string)  [unwired: 2 in, 8 out]
            n242 = Format Into String(format string=w740, w752) -> (resulting string=w751:string)  [unwired: 2 in, 1 out]
            n243 = call "Format Number for Table.vi"("Number"=w739) -> ("Number String"=w738:string)  [unwired: 2 in, 8 out]
            n244 = Format Into String(format string=w740, w750) -> (resulting string=w745:string)  [unwired: 2 in, 1 out]
            n245 = Format Into String(format string=w740, w749) -> (resulting string=w744:string)  [unwired: 2 in, 1 out]
            n246 = Format Into String(format string=w740, w748) -> (resulting string=w743:string)  [unwired: 2 in, 1 out]
            n247 = Format Into String(format string=w740, w747) -> (resulting string=w742:string)  [unwired: 2 in, 1 out]
            n248 = Format Into String(format string=w740, w746) -> (resulting string=w741:string)  [unwired: 2 in, 1 out]
            n249 = Format Into String(format string=w740, w738) -> (resulting string=w737:string)  [unwired: 2 in, 1 out]
          }
          n250 = Concatenate Strings(w549) -> (w543:string)
          n251 = Concatenate Strings(w548) -> (w542:string)
          n252 = Concatenate Strings(w547) -> (w538:string)
          n253 = Concatenate Strings(w546) -> (w541:string)
          n254 = Concatenate Strings(w545) -> (w540:string)
          n255 = Concatenate Strings(w544) -> (w539:string)
          n256 = Concatenate Strings(w501) -> (w500:string)
          n257 = Array Size(array=w510) -> (size(s)=w511:i32)
          n258 = Concatenate Strings(w510) -> (w550:string)
          n259 = call "Format Number for Table.vi"("Number"=w504) -> ("Number String"=w503:string)  [unwired: 2 in, 8 out]
          n260 = Increment(x=w511) -> (x+1=w509:i32)
          n261 = Format Into String(w509) -> (resulting string=w508:string)  [unwired: 3 in, 1 out]
          n262 = Format Into String(w512) -> (resulting string=w513:string)  [unwired: 3 in, 1 out]
          n263 = Format Into String(w515) -> (resulting string=w514:string)  [unwired: 3 in, 1 out]
        }
      }
      n264 = call "Keyed Array Add.vi"("case matching (sensitive)"=w30, "value"=w56, "key"="$$TEST_TYPE$$", "array in"=w35) -> ("array out"=w108:T2)  [unwired: 3 out]
      n265 = call "Keyed Array Add.vi"("case matching (sensitive)"=w30, "value"=w107, "key"="$$ALL_MEDIAN$$", "array in"=w108) -> ("array out"=w112:T2)  [unwired: 3 out]
      n266 = call "Keyed Array Add.vi"("case matching (sensitive)"=w30, "value"=w106, "key"="$$ALL_MEAN$$", "array in"=w112) -> ("array out"=w113:T2)  [unwired: 3 out]
      n267 = call "Keyed Array Add.vi"("case matching (sensitive)"=w30, "value"=w105, "key"="$$ALL_STD$$", "array in"=w113) -> ("array out"=w118:T2)  [unwired: 3 out]
      n268 = call "Keyed Array Add.vi"("case matching (sensitive)"=w30, "value"=w104, "key"="$$ALL_VAR$$", "array in"=w118) -> ("array out"=w119:T2)  [unwired: 3 out]
      n269 = call "Keyed Array Add.vi"("case matching (sensitive)"=w30, "value"=w103, "key"="$$ALL_MAX$$", "array in"=w119) -> ("array out"=w116:T2)  [unwired: 3 out]
      n270 = call "Keyed Array Add.vi"("case matching (sensitive)"=w30, "value"=w102, "key"="$$ALL_MIN$$", "array in"=w116) -> ("array out"=w54:T2)  [unwired: 3 out]
      n271 = call "Keyed Array Add.vi"("case matching (sensitive)"=w30, "value"=w52, "key"="$$ALL_N$$", "array in"=w54) -> ("array out"=w51:T2)  [unwired: 3 out]
      n272 = call "Keyed Array Add.vi"("value"=w62, "key"="$$freqtable$$", "array in"=w51) -> ("array out"=w64:T2)  [unwired: 1 in, 3 out]
      n273 = call "Keyed Array Add.vi"("case matching (sensitive)"=w30, "value"=w84, "key"="$$FREQ_ROW$$", "array in"=w64) -> ("array out"=w39:T2)  [unwired: 3 out]
      n274 = call "Keyed Array Add.vi"("case matching (sensitive)"=w30, "value"=w37, "key"="$$SHOWRAW$$", "array in"=w39) -> ("array out"=w38:T2)  [unwired: 3 out]
      n275 = call "Keyed Array Add.vi"("value"=w57, "key"="$$FREQ_COL$$", "array in"=w38) -> ("array out"=w80:T2)  [unwired: 1 in, 3 out]
      n276 = call "Keyed Array Add.vi"("case matching (sensitive)"=w30, "value"=w82, "key"="$$POINTS_ROW$$", "array in"=w80) -> ("array out"=w83:T2)  [unwired: 3 out]
      n277 = call "Keyed Array Add.vi"("case matching (sensitive)"=w30, "value"=w90, "key"="$$MEDIAN_ROW$$", "array in"=w83) -> ("array out"=w94:T2)  [unwired: 3 out]
      n278 = call "Keyed Array Add.vi"("case matching (sensitive)"=w30, "value"=w89, "key"="$$MEAN_ROW$$", "array in"=w94) -> ("array out"=w95:T2)  [unwired: 3 out]
      n279 = call "Keyed Array Add.vi"("case matching (sensitive)"=w30, "value"=w88, "key"="$$STD_ROW$$", "array in"=w95) -> ("array out"=w100:T2)  [unwired: 3 out]
      n280 = call "Keyed Array Add.vi"("case matching (sensitive)"=w30, "value"=w87, "key"="$$VAR_ROW$$", "array in"=w100) -> ("array out"=w101:T2)  [unwired: 3 out]
      n281 = call "Keyed Array Add.vi"("case matching (sensitive)"=w30, "value"=w86, "key"="$$MAX_ROW$$", "array in"=w101) -> ("array out"=w98:T2)  [unwired: 3 out]
      n282 = call "Keyed Array Add.vi"("case matching (sensitive)"=w30, "value"=w85, "key"="$$MIN_ROW$$", "array in"=w98) -> ("array out"=w50:T2)  [unwired: 3 out]
      n283 = call "Keyed Array Add.vi"("case matching (sensitive)"=w30, "value"=w47, "key"="$$N_ROW$$", "array in"=w50) -> ("array out"=w49:T2)  [unwired: 3 out]
      n284 = call "Keyed Array Add.vi"("case matching (sensitive)"=w30, "value"=w128, "key"="$$MEDIAN_COL$$", "array in"=w49) -> ("array out"=w138:T2)  [unwired: 3 out]
      n285 = call "Keyed Array Add.vi"("case matching (sensitive)"=w30, "value"=w125, "key"="$$MEAN_COL$$", "array in"=w138) -> ("array out"=w137:T2)  [unwired: 3 out]
      n286 = call "Keyed Array Add.vi"("case matching (sensitive)"=w30, "value"=w121, "key"="$$STD_COL$$", "array in"=w137) -> ("array out"=w126:T2)  [unwired: 3 out]
      n287 = call "Keyed Array Add.vi"("case matching (sensitive)"=w30, "value"=w124, "key"="$$VAR_COL$$", "array in"=w126) -> ("array out"=w120:T2)  [unwired: 3 out]
      n288 = call "Keyed Array Add.vi"("case matching (sensitive)"=w30, "value"=w123, "key"="$$MAX_COL$$", "array in"=w120) -> ("array out"=w132:T2)  [unwired: 3 out]
      n289 = call "Keyed Array Add.vi"("case matching (sensitive)"=w30, "value"=w122, "key"="$$MIN_COL$$", "array in"=w132) -> ("array out"=w46:T2)  [unwired: 3 out]
      n290 = call "Keyed Array Add.vi"("case matching (sensitive)"=w30, "value"=w44, "key"="$$N_COL$$", "array in"=w46) -> ("array out"=w45:T2)  [unwired: 3 out]
      n291 = call "Keyed Array Add.vi"("case matching (sensitive)"=w30, "value"=w67, "key"="$$#MNS$$", "array in"=w45) -> ("array out"=w68:T2)  [unwired: 3 out]
      n292 = call "Keyed Array Add.vi"("case matching (sensitive)"=w30, "value"=w129, "key"="$$MN_COL$$", "array in"=w68) -> ("array out"=w78:T2)  [unwired: 3 out]
      n293 = call "Keyed Array Add.vi"("case matching (sensitive)"=w30, "value"=w77, "key"="$$DETAIL_ROWS$$", "array in"=w78) -> ("array out"=w72:T2)  [unwired: 3 out]
      n294 = call "Keyed Array Add.vi"("case matching (sensitive)"=w30, "value"=w70, "key"="$$POINTS$$", "array in"=w72) -> ("array out"=w73:T2)  [unwired: 3 out]
      n295 = call "Keyed Array Add.vi"("case matching (sensitive)"=w30, "value"=w71, "key"="$$FREQS$$", "array in"=w73) -> ("array out"=w74:T2)  [unwired: 3 out]
      n296 = call "Keyed Array Add.vi"("case matching (sensitive)"=w30, "value"=w42, "key"="$$UNITS$$", "array in"=w74) -> ("array out"=w32:T2)  [unwired: 3 out]
      n297 = Concatenate Strings(w28, " ") -> (w27:string)
      n298 = Format Into String(initial string=w27, w29) -> (resulting string=w34:string)  [unwired: 2 in, 1 out]
      n299 = call "Keyed Array Add.vi"("case matching (sensitive)"=w30, "value"=w34, "key"="$$PROCESSED$$", "array in"=w32) -> ("array out"=w31:T2)  [unwired: 3 out]
    }
    frame 0, Default {
      w776 = Case_Matching."a == A" ("case matching (sensitive)")
      w771 = ""
      # "Measurement Name"
      # "Units"
      n300 = Unbundle By Name(w841) -> ("Test Type"=w796:string, "Sxx Format"=w845:string, "Parameter"=w846:string)  [unwired: 2 out]
      n301 = case shown="Default" w796 {
        tunnel: w798 -> [w857 w866]
        tunnel: [w857 w865] -> _
        tunnel: [w856 w862] -> w795
        tunnel: w797 -> [w856 w861]
        frame Default {
        }
        frame "PIM" {
          # "Is this a band edges case?"
          n302 = Index Array(array=w861) -> (element=w858:dbl)  [unwired: 1 in]
          n303 = for {
            tunnel: w858 -> [w869]
            tunnel: w861 -> [w868] mode=indexing
            tunnel: [w867] -> w860 mode=indexing
            n304 = Equal?(x=w869, y=w868) -> (x = y?=w867:bool)
          }
          n305 = Build Array(w858) -> (w863:dbl[])
          n306 = And Array Elements(Boolean array=w860) -> (logical AND=w859:bool)
          n307 = Select(t=0, s=w859, f=w866) -> (s? t:f=w865:i32)
          n308 = Select(t=w863, s=w859, f=w861) -> (s? t:f=w862:dbl[])
        }
      }
      n309 = Array Size(array=w795) -> ()  [unwired: 1 out]
      n310 = case shown="\"Prompted Inputs\", Default" w796 {
        tunnel: w845 -> [w872 _ _ _]
        tunnel: w846 -> [w870 w889 w895 w898]
        tunnel: [w874 w890 "dBm" ("search string") w899] -> w785
        tunnel: [w871 w889 w895 w898] -> w774
        tunnel: w770 -> [_ _ _ w897]
        frame "S Parameter" {
          n311 = case shown="\"Log Mag\", Default" w872 {
            tunnel: [T7."Log MAG" ("Display Format") T7."Lin MAG" ("Display Format") T7."VSWR" ("Display Format") T7."Phase" ("Display Format") T7."Delay" ("Display Format") T7."Insertion Loss" ("Display Format") T7."Isolation" ("Display Format") T7."Return Loss" ("Display Format")] -> w875
            frame "Log Mag", Default {
            }
            frame "Lin MAG" {
            }
            frame "VSWR" {
            }
            frame "Phase" {
            }
            frame "Delay" {
            }
            frame "Insertion Loss" {
            }
            frame "Isolation" {
            }
            frame "Return Loss" {
            }
          }
          n312 = Concatenate Strings(w870, " " ("search string"), w872) -> (w871:string)
          n313 = case shown="\"Log MAG\", \"Insertion Loss\"..\"Return Loss\", Default" w875 {
            tunnel: ["dB" "U" "x:1" "°" "s"] -> w874
            frame "Log MAG", "Insertion Loss".."Return Loss", Default {
            }
            frame "Lin MAG" {
            }
            frame "VSWR" {
            }
            frame "Phase" {
            }
            frame "Delay" {
            }
          }
        }
        frame "DC Attenuation" {
          n314 = Equal?(x=w889, y="Attenuation" ("search string")) -> (x = y?=w893:bool)
          n315 = Select(t="dB" ("search string"), s=w893, f="Ohm" ("search string")) -> (s? t:f=w890:string)
        }
        frame "PIM" {
        }
        frame "Prompted Inputs", Default {
          n316 = call "Fields Get Measurements.vi"("sDisplayName (empty, get all)"=w898, "Connection Refnum"=w897) -> ("Measurement Fields"=w901:T8[])  [unwired: 9 out]
          n317 = Index Array(array=w901) -> (element=w900:T8)  [unwired: 1 in]
          n318 = Unbundle By Name(w900) -> ("sUnits"=w899:string)
        }
      }
      n319 = call "Keyed Array Add.vi"("case matching (sensitive)"=w776, "value"=w796, "key"="$$TEST_TYPE$$", "array in"=w781) -> ("array out"=w826:T2)  [unwired: 3 out]
      n320 = call "Keyed Array Add.vi"("case matching (sensitive)"=w776, "value"=w771, "key"="$$ALL_MEDIAN$$", "array in"=w826) -> ("array out"=w830:T2)  [unwired: 3 out]
      n321 = call "Keyed Array Add.vi"("case matching (sensitive)"=w776, "value"=w771, "key"="$$ALL_MEAN$$", "array in"=w830) -> ("array out"=w831:T2)  [unwired: 3 out]
      n322 = call "Keyed Array Add.vi"("case matching (sensitive)"=w776, "value"=w771, "key"="$$ALL_STD$$", "array in"=w831) -> ("array out"=w836:T2)  [unwired: 3 out]
      n323 = call "Keyed Array Add.vi"("case matching (sensitive)"=w776, "value"=w771, "key"="$$ALL_VAR$$", "array in"=w836) -> ("array out"=w837:T2)  [unwired: 3 out]
      n324 = call "Keyed Array Add.vi"("case matching (sensitive)"=w776, "value"=w771, "key"="$$ALL_MAX$$", "array in"=w837) -> ("array out"=w834:T2)  [unwired: 3 out]
      n325 = call "Keyed Array Add.vi"("case matching (sensitive)"=w776, "value"=w771, "key"="$$ALL_MIN$$", "array in"=w834) -> ("array out"=w794:T2)  [unwired: 3 out]
      n326 = call "Keyed Array Add.vi"("case matching (sensitive)"=w776, "value"=w771, "key"="$$ALL_N$$", "array in"=w794) -> ("array out"=w792:T2)  [unwired: 3 out]
      n327 = call "Keyed Array Add.vi"("value"=w771, "key"="$$freqtable$$", "array in"=w792) -> ("array out"=w800:T2)  [unwired: 1 in, 3 out]
      n328 = call "Keyed Array Add.vi"("case matching (sensitive)"=w776, "value"=w771, "key"="$$FREQ_ROW$$", "array in"=w800) -> ("array out"=w784:T2)  [unwired: 3 out]
      n329 = call "Keyed Array Add.vi"("case matching (sensitive)"=w776, "value"=w771, "key"="$$SHOWRAW$$", "array in"=w784) -> ("array out"=w783:T2)  [unwired: 3 out]
      n330 = call "Keyed Array Add.vi"("value"=w771, "key"="$$FREQ_COL$$", "array in"=w783) -> ("array out"=w812:T2)  [unwired: 1 in, 3 out]
      n331 = call "Keyed Array Add.vi"("case matching (sensitive)"=w776, "value"=w771, "key"="$$POINTS_ROW$$", "array in"=w812) -> ("array out"=w814:T2)  [unwired: 3 out]
      n332 = call "Keyed Array Add.vi"("case matching (sensitive)"=w776, "value"=w771, "key"="$$MEDIAN_ROW$$", "array in"=w814) -> ("array out"=w818:T2)  [unwired: 3 out]
      n333 = call "Keyed Array Add.vi"("case matching (sensitive)"=w776, "value"=w771, "key"="$$MEAN_ROW$$", "array in"=w818) -> ("array out"=w819:T2)  [unwired: 3 out]
      n334 = call "Keyed Array Add.vi"("case matching (sensitive)"=w776, "value"=w771, "key"="$$STD_ROW$$", "array in"=w819) -> ("array out"=w824:T2)  [unwired: 3 out]
      n335 = call "Keyed Array Add.vi"("case matching (sensitive)"=w776, "value"=w771, "key"="$$VAR_ROW$$", "array in"=w824) -> ("array out"=w825:T2)  [unwired: 3 out]
      n336 = call "Keyed Array Add.vi"("case matching (sensitive)"=w776, "value"=w771, "key"="$$MAX_ROW$$", "array in"=w825) -> ("array out"=w822:T2)  [unwired: 3 out]
      n337 = call "Keyed Array Add.vi"("case matching (sensitive)"=w776, "value"=w771, "key"="$$MIN_ROW$$", "array in"=w822) -> ("array out"=w791:T2)  [unwired: 3 out]
      n338 = call "Keyed Array Add.vi"("case matching (sensitive)"=w776, "value"=w771, "key"="$$N_ROW$$", "array in"=w791) -> ("array out"=w790:T2)  [unwired: 3 out]
      n339 = call "Keyed Array Add.vi"("case matching (sensitive)"=w776, "value"=w771, "key"="$$MEDIAN_COL$$", "array in"=w790) -> ("array out"=w848:T2)  [unwired: 3 out]
      n340 = call "Keyed Array Add.vi"("case matching (sensitive)"=w776, "value"=w771, "key"="$$MEAN_COL$$", "array in"=w848) -> ("array out"=w847:T2)  [unwired: 3 out]
      n341 = call "Keyed Array Add.vi"("case matching (sensitive)"=w776, "value"=w771, "key"="$$STD_COL$$", "array in"=w847) -> ("array out"=w839:T2)  [unwired: 3 out]
      n342 = call "Keyed Array Add.vi"("case matching (sensitive)"=w776, "value"=w771, "key"="$$VAR_COL$$", "array in"=w839) -> ("array out"=w838:T2)  [unwired: 3 out]
      n343 = call "Keyed Array Add.vi"("case matching (sensitive)"=w776, "value"=w771, "key"="$$MAX_COL$$", "array in"=w838) -> ("array out"=w842:T2)  [unwired: 3 out]
      n344 = call "Keyed Array Add.vi"("case matching (sensitive)"=w776, "value"=w771, "key"="$$MIN_COL$$", "array in"=w842) -> ("array out"=w788:T2)  [unwired: 3 out]
      n345 = call "Keyed Array Add.vi"("case matching (sensitive)"=w776, "value"=w771, "key"="$$N_COL$$", "array in"=w788) -> ("array out"=w787:T2)  [unwired: 3 out]
      n346 = call "Keyed Array Add.vi"("case matching (sensitive)"=w776, "value"=w771, "key"="$$#MNS$$", "array in"=w787) -> ("array out"=w803:T2)  [unwired: 3 out]
      n347 = call "Keyed Array Add.vi"("case matching (sensitive)"=w776, "value"=w771, "key"="$$MN_COL$$", "array in"=w803) -> ("array out"=w810:T2)  [unwired: 3 out]
      n348 = call "Keyed Array Add.vi"("case matching (sensitive)"=w776, "value"=w771, "key"="$$DETAIL_ROWS$$", "array in"=w810) -> ("array out"=w805:T2)  [unwired: 3 out]
      n349 = call "Keyed Array Add.vi"("case matching (sensitive)"=w776, "value"=w771, "key"="$$POINTS$$", "array in"=w805) -> ("array out"=w806:T2)  [unwired: 3 out]
      n350 = call "Keyed Array Add.vi"("case matching (sensitive)"=w776, "value"=w771, "key"="$$FREQS$$", "array in"=w806) -> ("array out"=w807:T2)  [unwired: 3 out]
      n351 = call "Keyed Array Add.vi"("case matching (sensitive)"=w776, "value"=w785, "key"="$$UNITS$$", "array in"=w807) -> ("array out"=w778:T2)  [unwired: 3 out]
      n352 = Concatenate Strings(w774, " ") -> (w773:string)
      n353 = Format Into String(initial string=w773, w775) -> (resulting string=w780:string)  [unwired: 2 in, 1 out]
      n354 = call "Keyed Array Add.vi"("case matching (sensitive)"=w776, "value"=w780, "key"="$$PROCESSED$$", "array in"=w778) -> ("array out"=w777:T2)  [unwired: 3 out]
    }
  }
  "error out" <- w21
  "Keyed Array" <- w12
  "FORM" <- w2
  "columns" <- w1
